vi "open network for fast measurement.vi"(8 "error in (no error)":errorcluster, 10 "Data buffer size":i32, 11 "cRIO IP":string) -> (0 "error out":errorcluster, 1 "PCreaderV":refnum<k21>, 2 "PC para writer":refnum<k21>, 3 "PCreaderI":refnum<k21>)   [LabVIEW 2024]
uses:
  RT fast data.ctl
  <vilib>/LabVIEW Targets/FPGA/cRIO/shared/nicrio_ModuleControls/nicrio_cRIO-9775_RecordDataRates4ChansRing.ctl
  <vilib>/LabVIEW Targets/FPGA/cRIO/shared/nicrio_ModuleControls/nicrio_BasicConversionTime.ctl
  Ramps.ctl
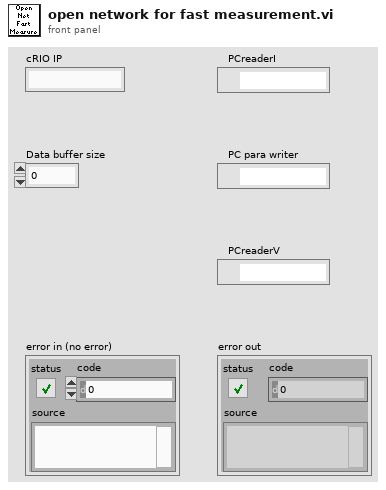
[diagram p1: front panel]
types:
  T1 = typedef "RT fast data.ctl" = cluster{"Records Num":i32, "AI Trigger Configuration":cluster{"Trigger Slope":enum8{"Positive", "Negative"}, "Trigger Level":fxp<+/-,17,5>, "Hystesis Value":fxp<+,16,4>, "AI Channel":u8}, "Record PreTrigger Samples":u32, "Record Samples":u32, "Ic Cut off or curve":bool, "Record Data Rate":T2, "Wait before trigger us":u32, "Cutoff delay usec":u32, "Timing Mode":T3, "Trigger length ticks":u32, "Timeout":i32, "Ramps":T4}
  T2 = typedef "nicrio_cRIO-9775_RecordDataRates4ChansRing.ctl" = u16
  T3 = typedef "nicrio_BasicConversionTime.ctl" = enum8{"High Speed", "High Resolution"}
  T4 = typedef "Ramps.ctl" = cluster{"Amp":fxp<+/-,20,5>, "Delay time 10us":i32, "Ramp1 time 10us":i32, "Ramp2 time 10us":i32, "Ramp3 time 10us":i32, "End time 10us":i32}
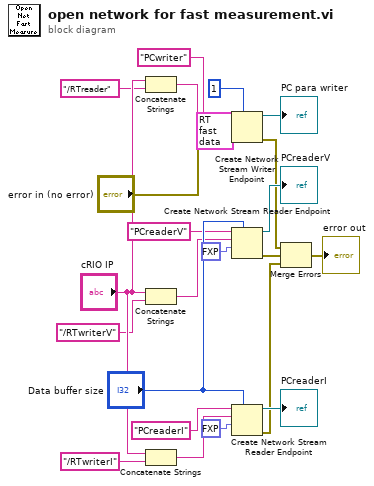
[diagram p0: block diagram]
diagram:
  n1 = Concatenate Strings("cRIO IP", "/RTreader" ("string")) -> (w4:string)
  n2 = Concatenate Strings("cRIO IP", "/RTwriterV" ("string")) -> (w11:string)
  n3 = Concatenate Strings("cRIO IP", "/RTwriterI" ("string")) -> (w17:string)
  n4 = Create Network Stream Writer Endpoint(7:1 ("writer buffer size"), 8:"error in (no error)", 9:T1 {"Records Num"=10000, "AI Trigger Configuration"={"Trigger Slope"=enum."Positive", "Trigger Level"=0.1298828125, "Hystesis Value"=0.0, "AI Channel"=0}, "Record PreTrigger Samples"=1, "Record Samples"=16, "Ic Cut off or curve"=TRUE, "Record Data Rate"=1, "Wait before trigger us"=10100, "Cutoff delay usec"=500, "Timing Mode"=enum."High Resolution", "Trigger length ticks"=15, "Timeout"=-1, "Ramps"={"Amp"=0.0, "Delay time 10us"=1, "Ramp1 time 10us"=1000, "Ramp2 time 10us"=2000, "Ramp3 time 10us"=1000, "End time 10us"=1}} ("Parameters"), 10:w4, 11:"PCwriter" ("writer name")) -> (0:w6:errorcluster, 3:→"PC para writer":refnum<k21>)  [unwired: 2 in]
  n5 = Create Network Stream Reader Endpoint(7:"Data buffer size", 9:fxp<+/-,17,5> 0.0, 10:w11, 11:"PCreaderV" ("reader name")) -> (0:w14:errorcluster, 3:→"PCreaderV":refnum<k21>)  [unwired: 3 in]
  n6 = Create Network Stream Reader Endpoint(7:"Data buffer size", 9:fxp<+/-,17,5> 0.0, 10:w17, 11:"PCreaderI" ("reader name")) -> (0:w19:errorcluster, 3:→"PCreaderI":refnum<k21>)  [unwired: 3 in]
  n7 = Merge Errors(w6, w14, w19) -> (→"error out":errorcluster)
